vi "Telegram Message Handler.vi"(8 "error in (no error)":errorcluster, 11 "Update":T1) -> (0 "error out":errorcluster)   [LabVIEW 2020, in "Notification.lvlib"]
uses:
  Notification.lvlib
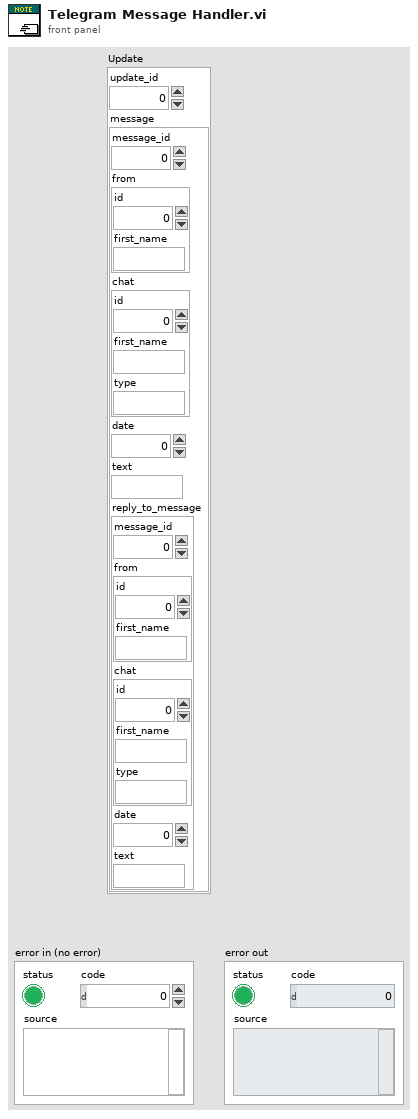
[diagram p1: front panel]
types:
  T1 = cluster{"update_id":u32, "message":cluster{"message_id":u32, "from":cluster{"id":u64, "first_name":string}, "chat":cluster{"id":i32, "first_name":string, "type":string}, "date":u32, "text":string, "reply_to_message":cluster{"message_id":u32, "from":cluster{"id":u64, "first_name":string}, "chat":cluster{"id":i32, "first_name":string, "type":string}, "date":u32, "text":string}}}
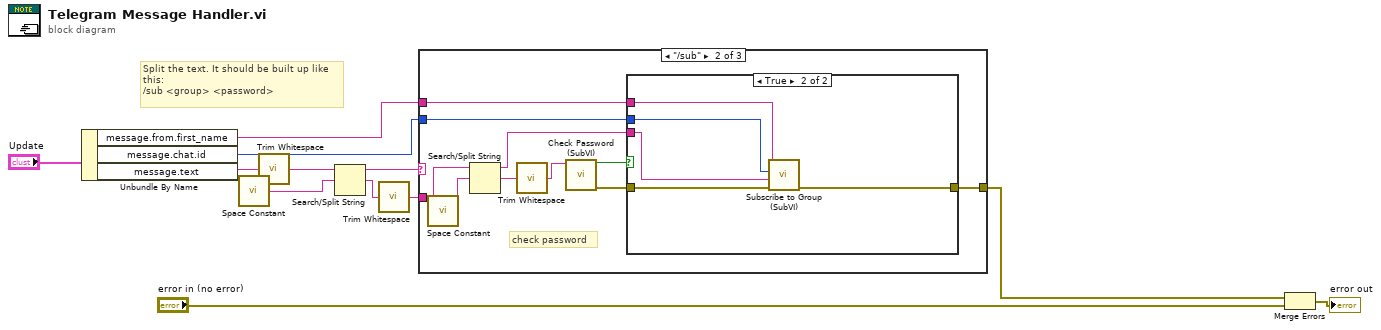
[diagram p0: block diagram]
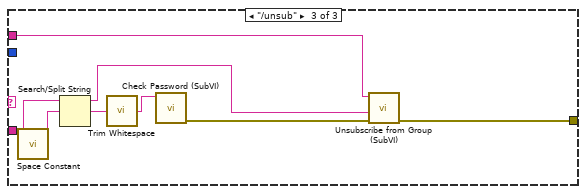
[diagram p4: hidden frame]
diagram:
  # "Split the text. It should be built up like\nthis:\n/sub <group> <password>"
  n1 = Unbundle By Name("Update") -> ("message.from.first_name"=w3:string, "message.chat.id"=w1:i32, "message.text"=w9:string)
  n2 = call <vilib>:"Space Constant.vi"() -> ("String"=w8:string)
  n3 = call <vilib>:"Trim Whitespace.vi"("string"=w9) -> ("trimmed string"=w4:string)  [unwired: 1 in]
  n4 = Search/Split String(string=w4, search string/char (-)=w8) -> (substring before match=w7:string, match + rest of string=w6:string)  [unwired: 1 in, 1 out]
  n5 = call <vilib>:"Trim Whitespace.vi"("string"=w6) -> ("trimmed string"=w5:string)  [unwired: 1 in]
  n6 = case shown="\"/sub\"" w7 {
    tunnel: w5 -> [_ w20 w35]
    tunnel: w3 -> [_ w15 w30]
    tunnel: [_ w14 w29] -> w2
    tunnel: w1 -> [_ w13 _]
    frame "False", Default {
    }
    frame "/sub" {
      # "check password"
      n7 = call <vilib>:"Space Constant.vi"() -> ("String"=w19:string)
      n8 = Search/Split String(string=w20, search string/char (-)=w19) -> (substring before match=w16:string, match + rest of string=w18:string)  [unwired: 1 in, 1 out]
      n9 = call <vilib>:"Trim Whitespace.vi"("string"=w18) -> ("trimmed string"=w17:string)  [unwired: 1 in]
      n10 = call "Check Password (SubVI).vi"("trimmed string"=w17) -> ("error out"=w21:errorcluster, "Checkbox"=w22:bool)  [unwired: 9 in]
      n11 = case shown="True" w22 {
        tunnel: w21 -> [w23 w28]
        tunnel: w16 -> [_ w26]
        tunnel: w15 -> [_ w24]
        tunnel: [w23 w27] -> w14
        tunnel: w13 -> [_ w25]
        frame False {
        }
        frame True {
          n12 = call "Subscribe to Group (SubVI).vi"("error in (no error)"=w28, "group"=w26, "chat id"=w25, "first_name"=w24) -> ("error out"=w27:errorcluster)  [unwired: 7 in]
        }
      }
    }
    frame "/unsub" {
      n13 = call <vilib>:"Space Constant.vi"() -> ("String"=w34:string)
      n14 = Search/Split String(string=w35, search string/char (-)=w34) -> (substring before match=w31:string, match + rest of string=w33:string)  [unwired: 1 in, 1 out]
      n15 = call <vilib>:"Trim Whitespace.vi"("string"=w33) -> ("trimmed string"=w32:string)  [unwired: 1 in]
      n16 = call "Check Password (SubVI).vi"("trimmed string"=w32) -> ("error out"=w36:errorcluster)  [unwired: 9 in, 1 out]
      n17 = call "Unsubscribe from Group (SubVI).vi"("error in (no error)"=w36, "group"=w31, "first_name"=w30) -> ("error out"=w29:errorcluster)  [unwired: 8 in]
    }
  }
  n18 = Merge Errors(w2, "error in (no error)") -> (→"error out":errorcluster)
